vi "仪器簇.vi"() -> ()   [LabVIEW 2020]
panel:
  in  "仪器地址7":T1
  in  "仪器地址6":T2
  in  "仪器地址5":T3
  in  "仪器地址4":T4
  in  "仪器地址3":T5
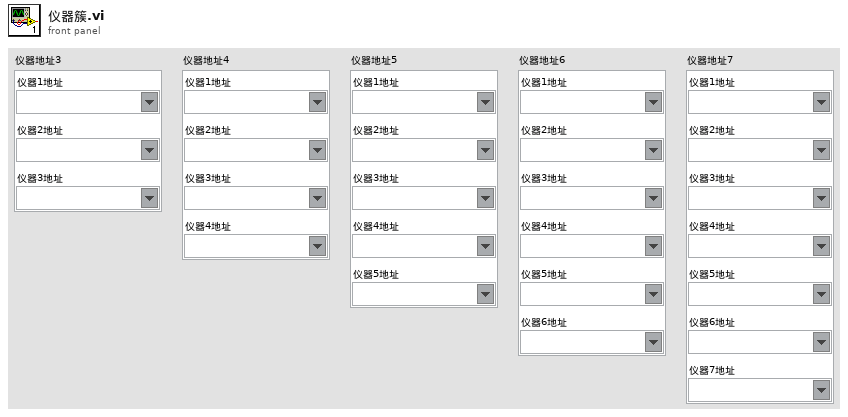
[diagram p1: front panel]
types:
  T1 = cluster{"仪器1地址":refnum<visa-resource-name>, "仪器2地址":refnum<visa-resource-name>, "仪器3地址":refnum<visa-resource-name>, "仪器4地址":refnum<visa-resource-name>, "仪器5地址":refnum<visa-resource-name>, "仪器6地址":refnum<visa-resource-name>, "仪器7地址":refnum<visa-resource-name>}
  T2 = cluster{"仪器1地址":refnum<visa-resource-name>, "仪器2地址":refnum<visa-resource-name>, "仪器3地址":refnum<visa-resource-name>, "仪器4地址":refnum<visa-resource-name>, "仪器5地址":refnum<visa-resource-name>, "仪器6地址":refnum<visa-resource-name>}
  T3 = cluster{"仪器1地址":refnum<visa-resource-name>, "仪器2地址":refnum<visa-resource-name>, "仪器3地址":refnum<visa-resource-name>, "仪器4地址":refnum<visa-resource-name>, "仪器5地址":refnum<visa-resource-name>}
  T4 = cluster{"仪器1地址":refnum<visa-resource-name>, "仪器2地址":refnum<visa-resource-name>, "仪器3地址":refnum<visa-resource-name>, "仪器4地址":refnum<visa-resource-name>}
  T5 = cluster{"仪器1地址":refnum<visa-resource-name>, "仪器2地址":refnum<visa-resource-name>, "仪器3地址":refnum<visa-resource-name>}
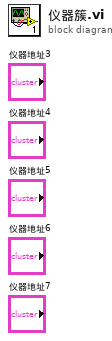
[diagram p0: block diagram]
diagram:
